vi "GlobalStop.vi"(2 "error in (no error)":errorcluster, 3 "Enum":enum16{"Clear", "Set", "Status"}(ring)) -> (0 "error out":errorcluster, 1 "Boolean":bool)   [LabVIEW 2023]
uses:
  <vilib>/rvi/Emulation/niFpgaGetClockAttributes.vi
  <vilib>/rvi/Emulation/niFpgaSctlEmulationGetInTimedLoop.vi
  <vilib>/rvi/Emulation/niFpgaEmulationReportErrorSimple.vi
  <vilib>/rvi/Emulation/niFpgaCriticalErrorInLSC.vi
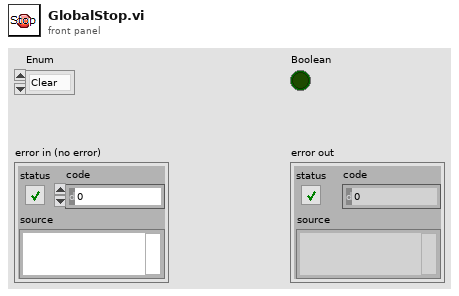
[diagram p1: front panel]
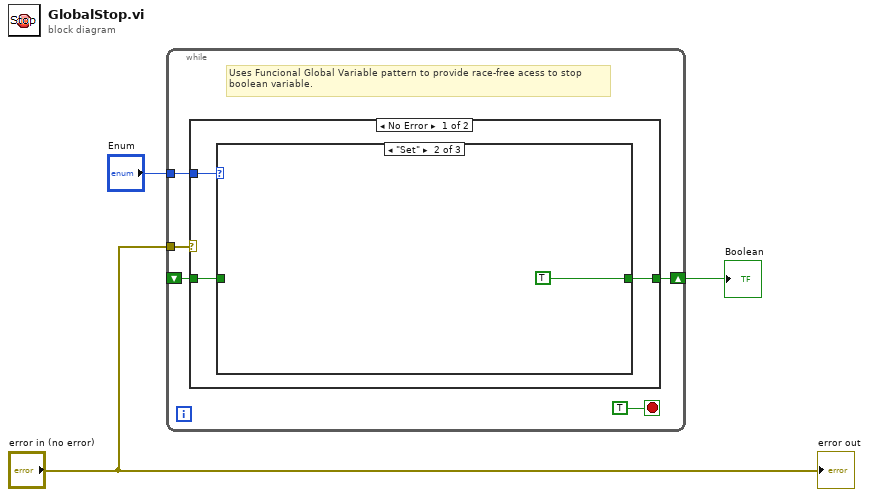
[diagram p0: block diagram]
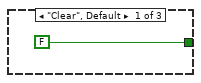
[diagram p2: hidden frame]
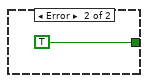
[diagram p4: hidden frame]
diagram:
  n1 = while {
    tunnel: "Enum" -> [w7]
    shift-right: [w6] -> w1
    shift-left: _ -> [w5]
    tunnel: "error in (no error)" -> [w4]
    stop <- TRUE stop-if-true
    # "Uses Funcional Global Variable pattern to provide race-free acess to stop\nboolean variable."
    n2 = case shown="No Error" w4 {
      tunnel: w7 -> [w11 _]
      tunnel: [w10 TRUE] -> w6
      tunnel: w5 -> [w9 _]
      frame No Error {
        n3 = case shown="\"Set\"" w11 {
          tunnel: [FALSE TRUE w14] -> w10
          tunnel: w9 -> [_ _ w14]
          frame "Clear", Default {
          }
          frame "Set" {
          }
          frame "Status" {
          }
        }
      }
      frame Error {
      }
    }
  }
  "Boolean" <- w1
  "error out" <- "error in (no error)"
